vi "lightfield normalization.vi"(10 "ROI array":u8[][](array[numeric])) -> (2 "ROI norm":sgl[][](array[numeric]))   [LabVIEW 2017]
uses:
  <vilib>/Analysis/NI_AALBase.lvlib
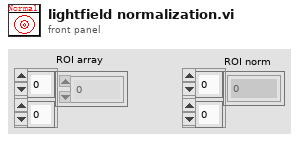
[diagram p1: front panel]
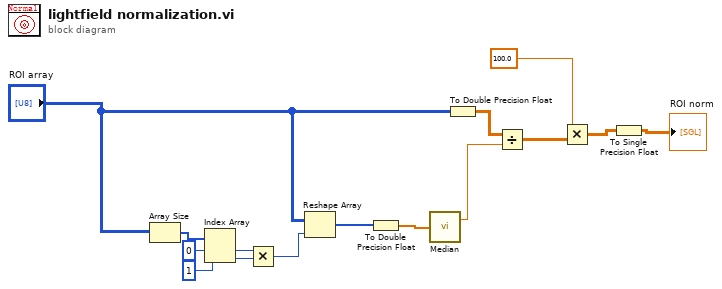
[diagram p0: block diagram]
diagram:
  n1 = Array Size(array="ROI array") -> (size(s)=w9:i32[])
  n2 = Index Array(array=w9, index #1=0 ("索引"), index #2=1 ("索引")) -> (element #1=w5:i32, element #2=w6:i32)
  n3 = Multiply(x=w5, y=w6) -> (x*y=w4:i32)
  n4 = Reshape Array("ROI array", w4) -> (w15:u8[])
  n5 = To Double Precision Float(number=w15) -> (double precision float=w14:dbl[])
  n6 = call <vilib>:"Median.vi"("X"=w14) -> ("median"=w13:dbl)  [unwired: 1 out]
  n7 = To Double Precision Float(number="ROI array") -> (double precision float=w12:dbl[][])
  n8 = Divide(x=w12, y=w13) -> (x/y=w10:dbl[][])
  n9 = Multiply(x=100.0, y=w10) -> (x*y=w2:dbl[][])
  n10 = To Single Precision Float(number=w2) -> (single precision float=→"ROI norm":sgl[][])
